vi "Write params.vi"(8 "error in (no error)":errorcluster, 10 "params JSON Tree In":variant, 11 "Request in":refnum<class "Request.lvclass">) -> (0 "error out":errorcluster, 3 "Request out":refnum<class "Request.lvclass">)   [LabVIEW 2015]
uses:
  params/params.lvclass
  Request.lvclass
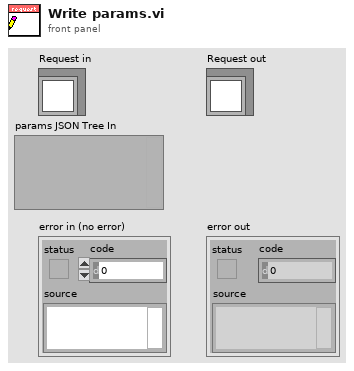
[diagram p1: front panel]
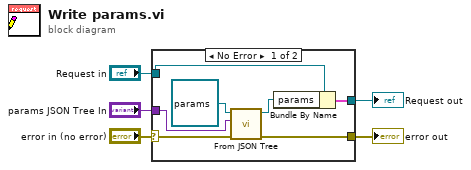
[diagram p0: block diagram]
diagram:
  n1 = case shown="No Error" "error in (no error)" {
    selector: "error in (no error)" -> [w8 w13]
    tunnel: [w7 w13] -> w4
    tunnel: [w11 w14] -> w2
    tunnel: "Request in" -> [w12 w14]
    tunnel: "params JSON Tree In" -> [w9 _]
    frame No Error {
      n2 = call-dynamic "From JSON Tree.vi"("error in (no error)"=w8, "JSON Tree In"=w9, "params in"=refnum<class "params.lvclass"> refnum ("params")) -> ("error out"=w7:errorcluster, "params out"=w6:refnum<class "params.lvclass">)  [unwired: 7 in]
      n3 = Bundle By Name(cluster=w12, "params"=w6) -> (w11:cluster{})
    }
    frame Error {
    }
  }
  "error out" <- w4
  "Request out" <- w2
